vi "Get Auto Box.vi"() -> (0 "Shoot During Autonomous?":bool, 1 "Use Hot Goal?":bool, 2 "2 Ball Autonomous?":bool)   [LabVIEW 2013]
uses:
  <vilib>/Rock Robotics/WPI/DigitalInput/WPI_DigitalInputDevRef.ctl
  <vilib>/Rock Robotics/SystemInterfaces/DIO/FPGA_DIOChannel.ctl
  <vilib>/Rock Robotics/SystemInterfaces/Typedef/FPGA_TypedefDigitalModule.ctl
  typedefs/fg_typedef.ctl
panel:
  # "Read the Autonomous Switch Box to Determine what Autonomous Does"
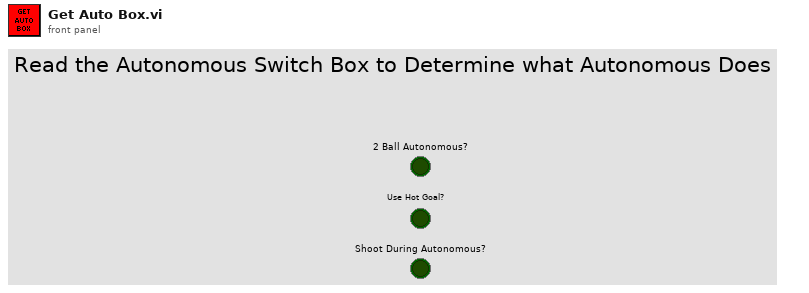
[diagram p1: front panel]
types:
  T1 = typedef "WPI_DigitalInputDevRef.ctl" = cluster{"DevStatus":errorcluster, "DIO Channel":T2, "Digital Module":T3}
  T2 = typedef "FPGA_DIOChannel.ctl" = enum8{"DIO 1", "DIO 2", "DIO 3", "DIO 4", "DIO 5", "DIO 6", "DIO 7", "DIO 8", "DIO 9", "DIO 10", "DIO 11", "DIO 12", "DIO 13", "DIO 14", "Invalid"}
  T3 = typedef "FPGA_TypedefDigitalModule.ctl" = enum16{"Digital Module 1", "Digital Module 2"}
  T4 = typedef "fg_typedef.ctl" = enum16{"Get", "Set"}
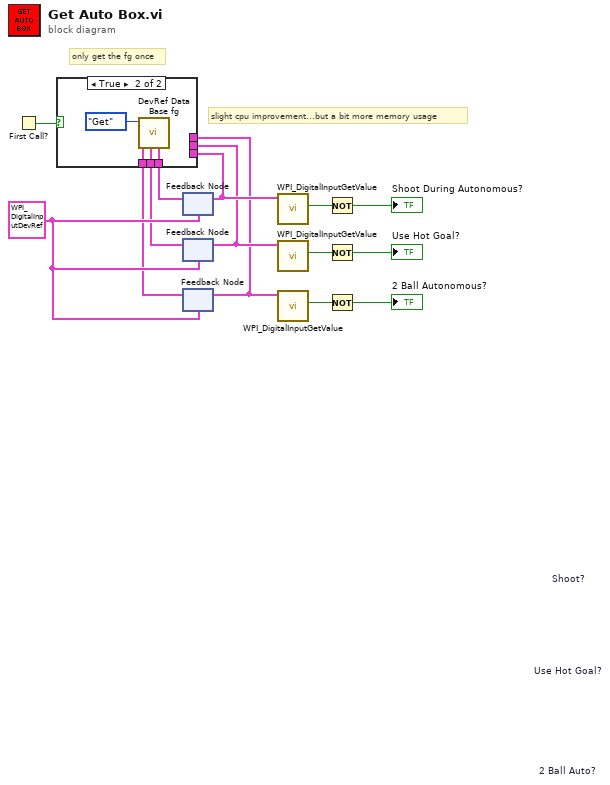
[diagram p0: block diagram]
diagram:
  w13 = T1 {"DevStatus"={"status"=FALSE, "code"=0, "source"=""}, "DIO Channel"=enum."DIO 1", "Digital Module"=enum."Digital Module 1"} ("2ball")
  # "slight cpu improvement...but a bit more memory usage"
  # "only get the fg once"
  n1 = First Call?() -> (First Call?: T/F=w14:bool)
  n2 = feedback #1 "Shoot?"(w13) -> (w9:T1)
  n3 = feedback #2 "Use Hot Goal?"(w13) -> (w6:T1)
  n4 = feedback #3 "2 Ball Auto?"(w13) -> (w2:T1)
  n5 = case shown="True" w14 {
    tunnel: [w17 w20] -> w12
    tunnel: [w16 w19] -> w11
    tunnel: [w15 w18] -> w10
    tunnel: w9 -> [w17 _]
    tunnel: w6 -> [w16 _]
    tunnel: w2 -> [w15 _]
    frame False {
    }
    frame True {
      n6 = call "DevRef Data Base fg.vi"("Menu"=fg_typedef."Get") -> ("autoshoot"=w20:T1, "hotgoal"=w19:T1, "2ball"=w18:T1)  [unwired: 2 in, 6 out]
    }
  }
  n7 = feedback-in #1(w12) -> ()
  n8 = feedback-in #2(w11) -> ()
  n9 = feedback-in #3(w10) -> ()
  n10 = call <vilib>:"WPI_DigitalInputGetValue.vi"("DigitalInputDevRef"=w9) -> ("Value"=w8:bool)  [unwired: 8 in, 2 out]
  n11 = call <vilib>:"WPI_DigitalInputGetValue.vi"("DigitalInputDevRef"=w6) -> ("Value"=w5:bool)  [unwired: 8 in, 2 out]
  n12 = call <vilib>:"WPI_DigitalInputGetValue.vi"("DigitalInputDevRef"=w2) -> ("Value"=w3:bool)  [unwired: 8 in, 2 out]
  n13 = Not(x=w8) -> (.not. x?=→"Shoot During Autonomous?":bool)
  n14 = Not(x=w5) -> (.not. x?=→"Use Hot Goal?":bool)
  n15 = Not(x=w3) -> (.not. x?=→"2 Ball Autonomous?":bool)
